vi "Leak Actor State.vi"(8 "error in (no error)":errorcluster, 10 "Location":T1=enum."Stop Core", 11 "ViewableOne in":refnum<class "LeakyViewable.lvclass">) -> (0 "error out":errorcluster, 3 "ViewableOne out":refnum<class "LeakyViewable.lvclass">)   [LabVIEW 2017, in "LeakyViewable.lvlib" / "LeakyViewable.lvclass"]
uses:
  LeakyViewable.lvclass
  c:/Git/mva-viewable/Source/IViewable/IViewable/IViewable.lvclass
  Leak Location.ctl
  LeakyViewable.lvclass/LeakyViewable.ctl
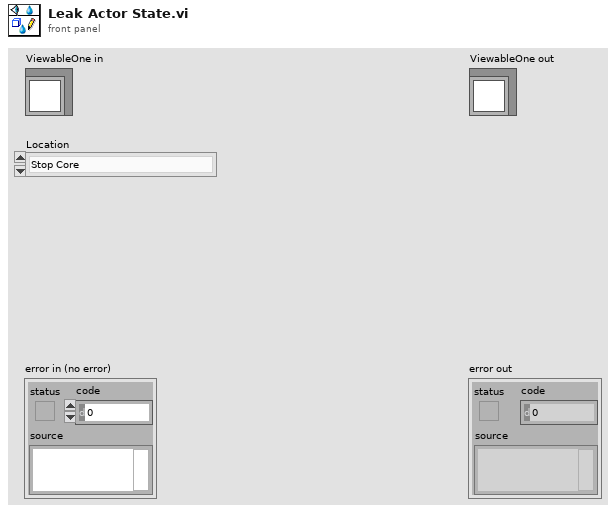
[diagram p1: front panel]
types:
  T1 = typedef "LeakyViewable.lvlib/LeakyViewable.lvclass/Leak Location.ctl" = enum16{"Pre Launch Init", "Entering Actor Core", "Actor Core", "Exiting Actor Core", "Stop Core", "Handle Error"}
  T2 = cluster{"Location":T1, "ViewableOne in":refnum<class "LeakyViewable.lvclass">, "error in (no error)":errorcluster}
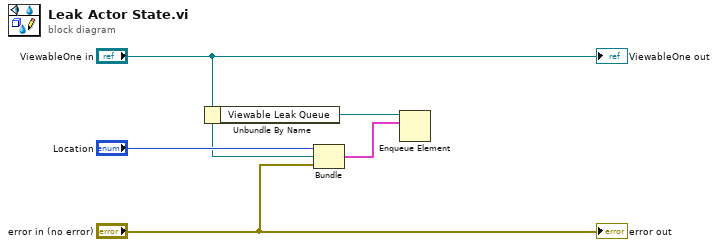
[diagram p0: block diagram]
diagram:
  n1 = Unbundle By Name("ViewableOne in") -> ("Viewable Leak Queue"=w5:refnum<queue>)
  n2 = Bundle("Location"="Location", "ViewableOne in"="ViewableOne in", "error in (no error)"="error in (no error)") -> (w4:T2)  [unwired: 1 in]
  n3 = Enqueue Element(queue=w5, element=w4) -> ()  [unwired: 2 in, 3 out]
  "error out" <- "error in (no error)"
  "ViewableOne out" <- "ViewableOne in"
